vi "generate classes from ini.vi"   [LabVIEW 2020]
uses:
  <vilib>/Utility/config.llb/Read Key (String).vi
  <vilib>/Utility/config.llb/NI_LVConfig.lvlib
  <vilib>/Utility/miscctls.llb/LVPointTypeDef.ctl
types:
  T1 = typedef "NI_LVConfig.lvlib/Config Data RefNum.ctl" = refnum<k1>
  T2 = typedef "LVPointTypeDef.ctl" = cluster{"Horizontal":i16, "Vertical":i16}
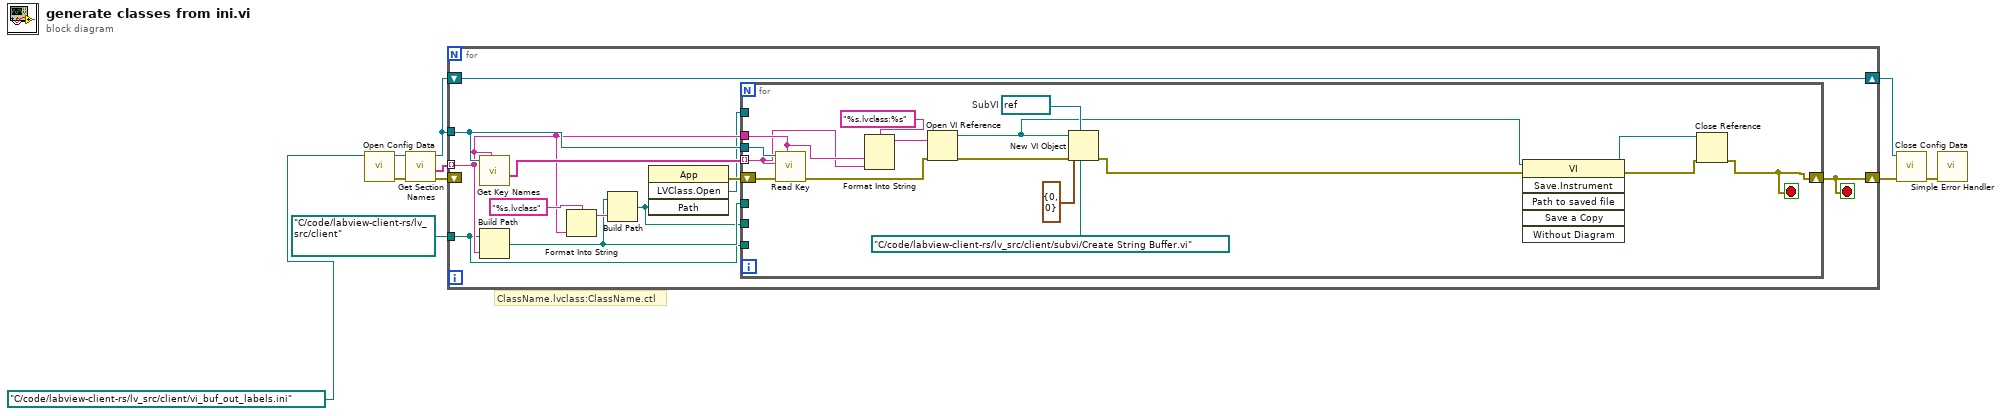
[diagram p0: block diagram]
diagram:
  # "ClassName.lvclass:ClassName.ctl"
  n1 = call <vilib>:"Open Config Data.vi"("configuration file path"=path "C:/code/labview-client-rs/lv_src/client/vi_buf_out_labels.ini") -> ("error out"=w5:errorcluster, "refnum"=w10:T1)  [unwired: 8 in, 1 out]
  n2 = call <vilib>:"Get Section Names.vi"("error in (no error)"=w5, "refnum"=w10) -> ("error out"=w7:errorcluster, "section names"=w9:string[], "refnum out"=w2:T1)  [unwired: 7 in]
  n3 = for {
    tunnel: w9 -> [w16] mode=indexing
    shift-right: [w22] -> w8
    shift-left: w2 -> [w22]
    shift-right: [w12] -> w6
    shift-left: w7 -> [_]
    tunnel: path "C:/code/labview-client-rs/lv_src/client" ("Path") -> [w13]
    tunnel: w2 -> [w18]
    stop <- w12 stop-if-true
    n4 = call <vilib>:"Get Key Names.vi"("section"=w16, "refnum"=w18) -> ("key names"=w17:string[])  [unwired: 6 in, 3 out]
    n5 = Build Path(base path=w13, name or relative path=w16) -> (appended path=w19:path)
    n6 = Format Into String(format string="%s.lvclass", w16) -> (resulting string=w20:string)  [unwired: 2 in, 1 out]
    n7 = Build Path(base path=w19, name or relative path=w20) -> (appended path=w11:path)
    n8 = invoke class="App" method="LVClass.Open"("Path"=w11) -> (error out=w15:errorcluster, "LVClass.Open"=w14:refnum<vi>)  [unwired: 3 in, 2 out]
    n9 = for {
      tunnel: w19 -> [_]
      tunnel: w18 -> [w37]
      tunnel: w17 -> [w29] mode=indexing
      tunnel: w16 -> [w33]
      tunnel: w14 -> [_]
      tunnel: w13 -> [_]
      shift-right: [w30] -> w12
      shift-left: w15 -> [w38]
      tunnel: w11 -> [_]
      stop <- w30 stop-if-true
      w27 = refnum<vi> refnum  # SubVI
      n10 = call-poly <vilib>:"Read Key.vi"("section"=w33, "error in (no error)"=w38, "key"=w29, "refnum"=w37) -> ("error out"=w34:errorcluster)  [unwired: 4 in, 3 out]
      n11 = Format Into String(format string="%s.lvclass:%s", w33, w29) -> (resulting string=w35:string)  [unwired: 2 in, 1 out]
      n12 = Open VI Reference(vi path=w35, error in (no error)=w34) -> (vi reference=w23:refnum<vi>, error out=w25:errorcluster)  [unwired: 4 in]
      n13 = New VI Object(vi object class=w27, owner refnum=w23, position/next to=T2 {"Horizontal"=0, "Vertical"=0} ("location"), 6:path "C:/code/labview-client-rs/lv_src/client/subvi/Create String Buffer.vi" ("path"), 8:w25) -> (0:w24:errorcluster)  [unwired: 3 in, 1 out]
      n14 = invoke class="VI" method="Save.Instrument"(reference=w23, error in=w24) -> (reference out=w32:refnum<vi>, error out=w31:errorcluster)  [unwired: 4 in, 4 out]
      n15 = Close Reference(reference=w32, error in (no error)=w31) -> (error out=w30:errorcluster)
    }
  }
  n16 = call <vilib>:"Close Config Data.vi"("error in (no error)"=w6, "refnum"=w8) -> ("error out"=w4:errorcluster)  [unwired: 8 in, 1 out]
  n17 = call <vilib>:"Simple Error Handler.vi"("error in (no error)"=w4) -> ()  [unwired: 4 in, 5 out]
